vi "install_core.vi"(11 "CLI":path) -> (2 "Comando_Compile":string)   [LabVIEW 2025]
doc: "VI para compilar el firmware usando Arduino CLI"
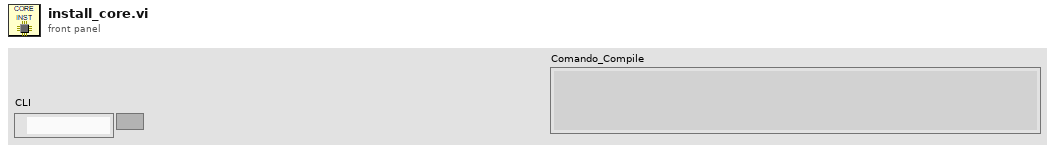
[diagram p1: front panel]
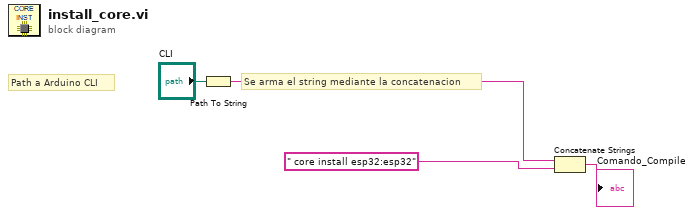
[diagram p0: block diagram]
diagram:
  # "Se arma el string mediante la concatenacion"
  # "Path a Arduino CLI"
  n1 = Path To String(path="CLI") -> (string=w3:string)
  n2 = Concatenate Strings(w3, " core install esp32:esp32" ("string")) -> (→"Comando_Compile":string)
